vi "Create PDFDocument.vi"(0 "PDF Report IN":refnum<class "PDF Report Class.lvclass">, 2 "Open or create":T1, 11 "error in (no error)":errorcluster) -> (4 "PDF Report OUT":refnum<class "PDF Report Class.lvclass">, 15 "error out":errorcluster)   [LabVIEW 2019, in "Exaprom PDF.lvlib"]
doc: "Version 1.1\nDeveloped by Jean-Marc Simard\nCopyright © 2012, Exaprom Inc.\nAll rights reserved.\nLicense: BSD\n\nWith iTextSharp 4.1.6 (http://itextsharp.sourceforge.net)\nunder Mozilla Public License Version 1.1\n(http://www.mozilla.org/MPL/MPL-1.1.html)"
uses:
  LV Class/PDF Report Class/PDF Report Class.lvclass
  Controls/General Controls/Create, open or close.ctl
  C:/work/niobrara_lv/labview pdf writer fixing/DLL/itextsharp.dll
  DLL/itextsharp.dll
  Exaprom PDF.lvlib
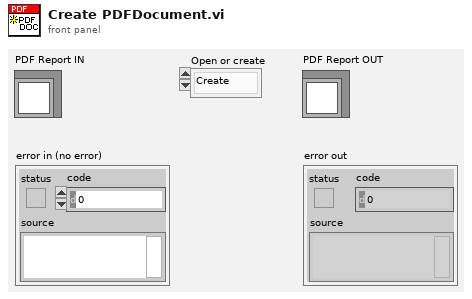
[diagram p1: front panel]
types:
  T1 = typedef "Exaprom PDF.lvlib/Create, open or close.ctl" = enum16{"Create", "Open", "Close"}
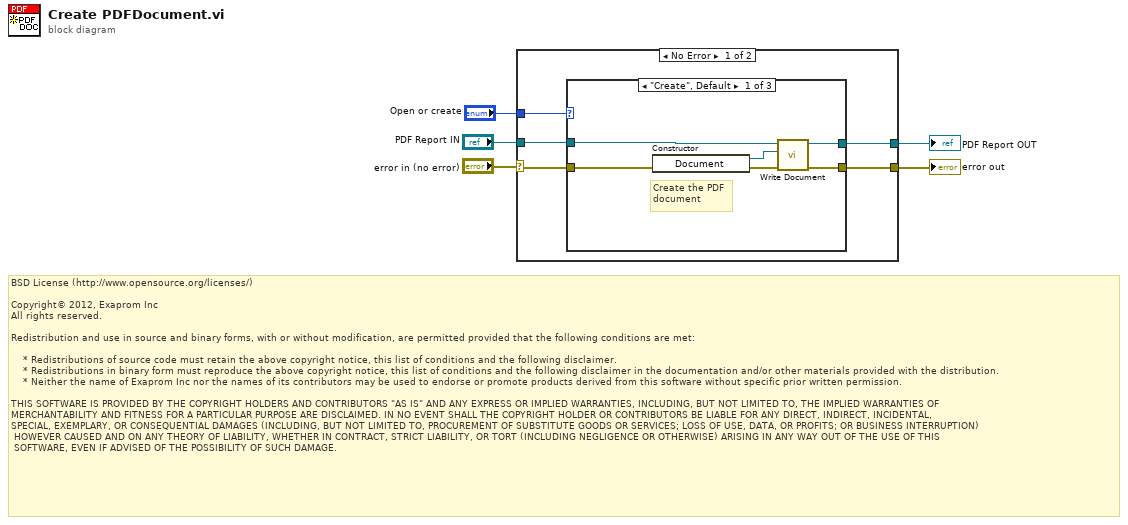
[diagram p0: block diagram]
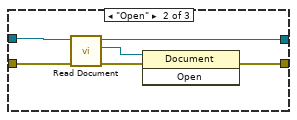
[diagram p2: hidden frame]
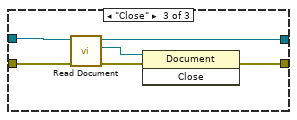
[diagram p3: hidden frame]
diagram:
  # "BSD License (http://www.opensource.org/licenses/)\n\nCopyright© 2012, Exaprom Inc\nAll rights reserved.\n\nRedistribution and use in source and binary forms, with or without modification, are permitted provided that the following conditions are met:\n\n    * Redistributions of source code must retain the above copyright notice, this list of conditions and the following disclaimer.\n    * Redistributions in binary form must reproduce the above copyright notice, this list of conditions and the following disclaimer in the documentation and/or other materials provided with the distribution.\n    * Neither the name of Exaprom Inc nor the names of its contributors may be used to endorse or promote products derived from this software without specific prior written permission.\n\nTHIS SOFTWARE IS PROVIDED BY THE COPYRIGHT HOLDERS AND CONTRIBUTORS \"AS IS\" AND ANY EXPRESS OR IMPLIED WARRANTIES, INCLUDING, BUT NOT LIMITED TO, THE IMPLIED WARRANTIES OF \nMERCHANTABILITY AND FITNESS FOR A PARTICULAR PURPOSE ARE DISCLAIMED. IN NO EVENT SHALL THE COPYRIGHT HOLDER OR CONTRIBUTORS BE LIABLE FOR ANY DIRECT, INDIRECT, INCIDENTAL,\nSPECIAL, EXEMPLARY, OR CONSEQUENTIAL DAMAGES (INCLUDING, BUT NOT LIMITED TO, PROCUREMENT OF SUBSTITUTE GOODS OR SERVICES; LOSS OF USE, DATA, OR PROFITS; OR BUSINESS INTERRUPTION)\n HOWEVER CAUSED AND ON ANY THEORY OF LIABILITY, WHETHER IN CONTRACT, STRICT LIABILITY, OR TORT (INCLUDING NEGLIGENCE OR OTHERWISE) ARISING IN ANY WAY OUT OF THE USE OF THIS\n SOFTWARE, EVEN IF ADVISED OF THE POSSIBILITY OF SUCH DAMAGE."
  n1 = case shown="No Error" "error in (no error)" {
    selector: "error in (no error)" -> [w7 w30]
    tunnel: "PDF Report IN" -> [w9 w29]
    tunnel: [w8 w29] -> w4
    tunnel: [w6 w30] -> w3
    tunnel: "Open or create" -> [w10 _]
    frame No Error {
      n2 = case shown="\"Create\", Default" w10 {
        tunnel: w9 -> [w14 w21 w27]
        tunnel: [w13 w17 w23] -> w8
        tunnel: w7 -> [w12 w22 w28]
        tunnel: [w11 w18 w24] -> w6
        frame "Create", Default {
          # "Create the PDF\ndocument"
          n3 = constructor class="Document"(error in=w12) -> (reference out=w16:refnum<k24>, error out=w15:errorcluster)  [unwired: 2 in, 1 out]
          n4 = call-dynamic "Write Document.vi"("error in (no error)"=w15, "Document"=w16, "PDF Report Class in"=w14) -> ("error out"=w11:errorcluster, "PDF Report Class out"=w13:refnum<class "PDF Report Class.lvclass">)  [unwired: 7 in]
        }
        frame "Open" {
          n5 = call-dynamic "Read Document.vi"("error in (no error)"=w22, "PDF Report Class in"=w21) -> ("error out"=w20:errorcluster, "Document"=w19:refnum<k24>, "PDF Report Class out"=w17:refnum<class "PDF Report Class.lvclass">)  [unwired: 7 in]
          n6 = invoke class="Document" method="Open"(reference=w19, error in=w20) -> (error out=w18:errorcluster)  [unwired: 1 in, 2 out]
        }
        frame "Close" {
          n7 = call-dynamic "Read Document.vi"("error in (no error)"=w28, "PDF Report Class in"=w27) -> ("error out"=w26:errorcluster, "Document"=w25:refnum<k24>, "PDF Report Class out"=w23:refnum<class "PDF Report Class.lvclass">)  [unwired: 7 in]
          n8 = invoke class="Document" method="Close"(reference=w25, error in=w26) -> (error out=w24:errorcluster)  [unwired: 1 in, 2 out]
        }
      }
    }
    frame Error {
    }
  }
  "PDF Report OUT" <- w4
  "error out" <- w3
